vi "Average Sector Data.vi"() -> ()   [LabVIEW 2013]
panel:
  in  "Sector Edges":u8[][](array[numeric])
  in  "[Average Sector Data] Test":u8[][](array[numeric])
  in  "[Average Sector Data]":u8[](array[numeric])
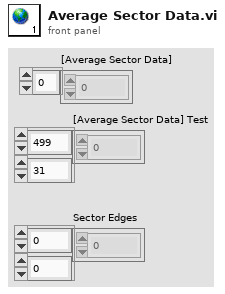
[diagram p1: front panel]
diagram:
